vi "V1_moveby_commands_all.vi"(8 "error in (no error)":errorcluster, 9 "DAQ channel":tag, 10 "channel":i32(ring)=1 items=["Channel1"=1, "Channel2"=2, "Channel3"=3, "Channel4"=4], 11 ".NET Refnum in":refnum<k24>) -> (0 "error out":errorcluster, 3 ".NET Refnum out":refnum<k24>)   [LabVIEW 2020]
uses:
  C:/Users/359167/Documents/LabVIEW_ws/Thorlabs.MotionControl.KCube.InertialMotorCLI.dll
  Thorlabs.MotionControl.KCube.InertialMotorCLI.dll
  <vilib>/DAQmx/read.llb/DAQmx Read (Analog 1D Wfm NChan NSamp).vi
  <vilib>/Analysis/baseanly.llb/Mean (DBL).vi
  <vilib>/DAQmx/create/channels.llb/DAQmx Create Channel (AI-Voltage-Basic).vi
  <vilib>/DAQmx/configure/timing.llb/DAQmx Timing (Sample Clock).vi
  <vilib>/DAQmx/miscellaneous.llb/DAQmx Fill In Error Info.vi
  <vilib>/Analysis/NI_AALBase.lvlib
panel:
  out "x*y":dbl
  out "Sensor Sampling":waveform(dbl)[](graph)
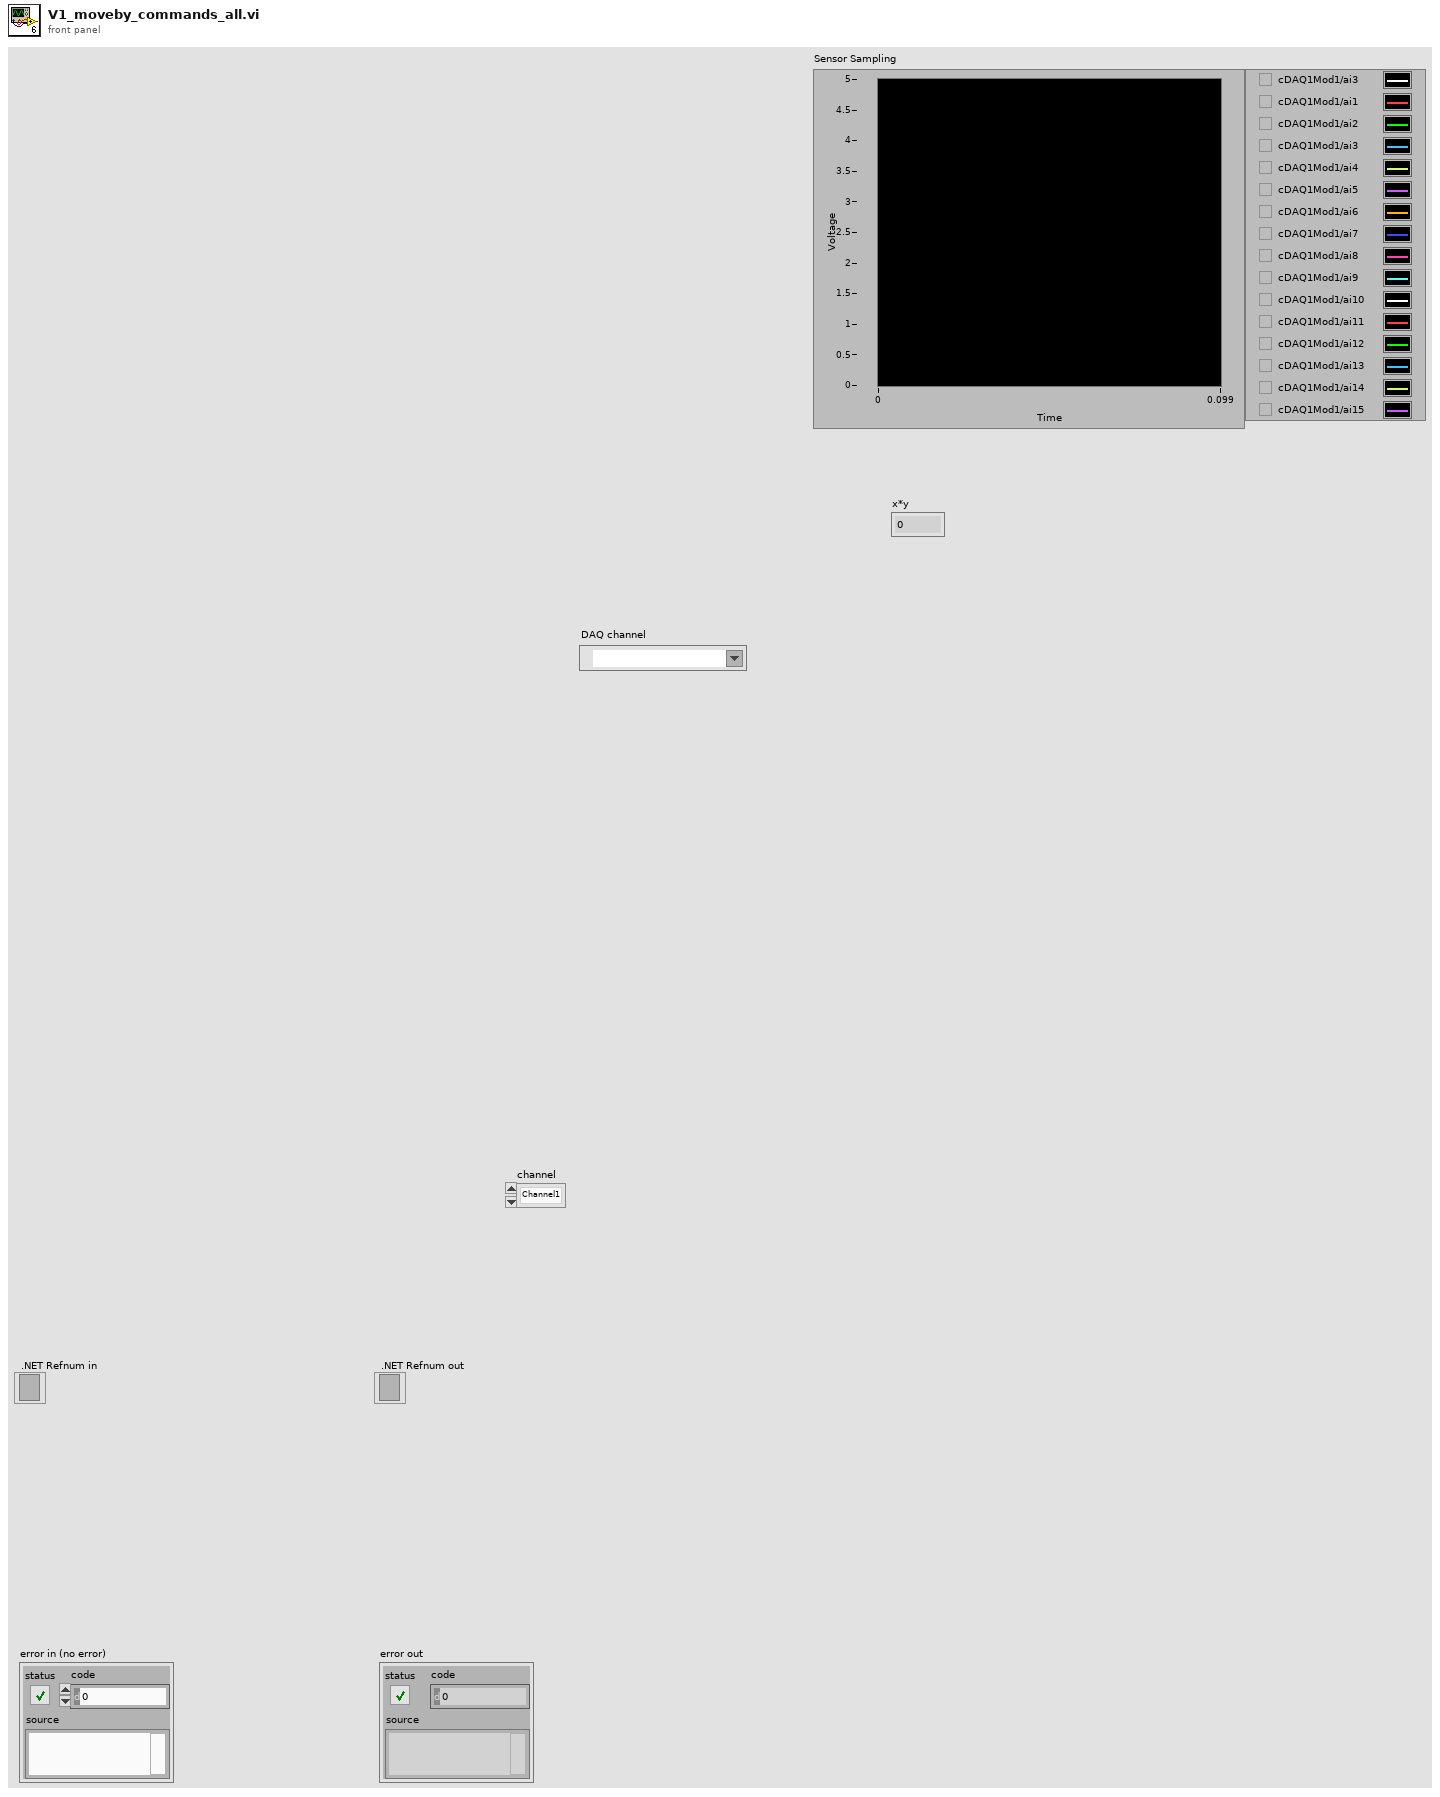
[diagram p1: front panel]
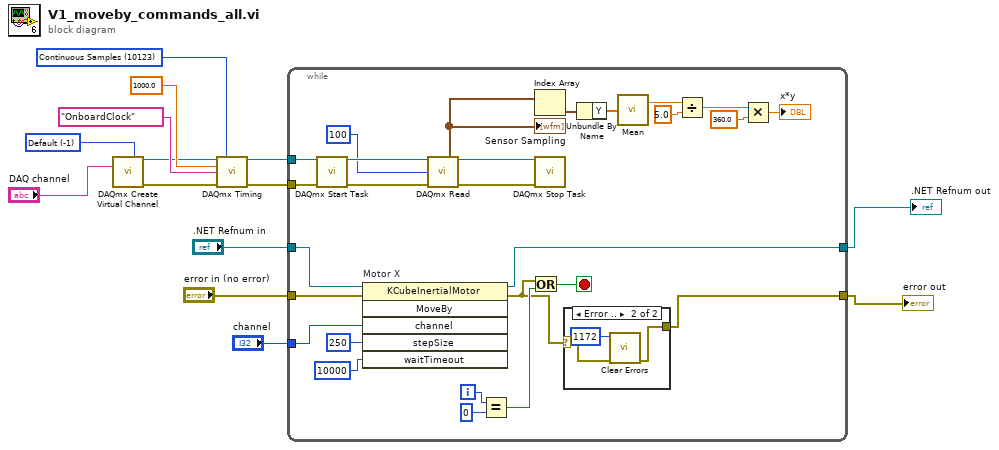
[diagram p0: block diagram]
diagram:
  w10 = -1 items=["Default"=-1, "RSE"=10083, "NRSE"=10078, "Differential"=10106, "Pseudodifferential"=12529] ("input terminal configuration")
  w11 = 10123 items=["Finite Samples"=10178, "Continuous Samples"=10123, "Hardware Timed Single Point"=12522] ("sample mode")
  n1 = call-poly <vilib>:"DAQmx Create Virtual Channel.vi"("input terminal configuration"=w10, "physical channels"="DAQ channel") -> ("task out"=w6:refnum<k21>, "error out"=w7:errorcluster)  [unwired: 12 in]
  n2 = call-poly <vilib>:"DAQmx Timing.vi"("task/channels in"=w6, "sample mode"=w11, "rate"=1000.0 ("sample rate"), "source"=tag "OnboardClock", "error in"=w7) -> ("task out"=w4:refnum<k21>, "error out"=w3:errorcluster)  [unwired: 9 in]
  n3 = while {
    tunnel: "channel" -> [w39]
    tunnel: w4 -> [w19]
    tunnel: w3 -> [w18]
    tunnel: ".NET Refnum in" -> [w33]
    tunnel: [w17] -> w1
    tunnel: "error in (no error)" -> [w37]
    tunnel: [w15] -> w2
    i -> [w34]
    stop <- w35 stop-if-true
    n4 = call <vilib>:"DAQmx Start Task.vi"("task/channels in"=w19, "error in"=w18) -> ("task out"=w29:refnum<k21>, "error out"=w30:errorcluster)  [unwired: 12 in]
    n5 = invoke on="Motor X" class="KCubeInertialMotor" method="MoveBy"(reference=w33, error in=w37, "channel"=w39, "stepSize"=250, "waitTimeout"=10000) -> (reference out=w17:refnum<k24>, error out=w16:errorcluster)  [unwired: 1 in, 4 out]
    n6 = call-poly <vilib>:"DAQmx Read.vi"("task/channels in"=w29, "number of samples per channel"=100 ("n samples/channel"), "error in"=w30) -> ("data"=w21:waveform(dbl)[], "task out"=w31:refnum<k21>, "error out"=w32:errorcluster)  [unwired: 10 in]
    "Sensor Sampling" <- w21
    n7 = Equal?(x=w34, y=0) -> (x = y?=w36:bool)
    n8 = Or(x=w16, y=w36) -> (x .or. y?=w35:bool)
    n9 = Index Array(array=w21) -> (element=w27:waveform(dbl))  [unwired: 1 in]
    n10 = call <vilib>:"DAQmx Stop Task.vi"("task/channels in"=w31, "error in"=w32) -> ()  [unwired: 12 in, 2 out]
    n11 = case shown="Error .." w16 {
      selector: w16 -> [w42 w44]
      tunnel: [w42 w43] -> w15
      frame No Error {
      }
      frame Error {
        n12 = call <vilib>:"Clear Errors.vi"("error in (no error)"=w44, "specific error code to clear (0: all)"=1172) -> ("error out"=w43:errorcluster)  [unwired: 4 in, 1 out]
      }
    }
    n13 = Unbundle By Name(w27) -> ("Y"=w26:dbl[])
    n14 = call-poly <vilib>:"Mean.vi"("X"=w26) -> ("mean"=w25:dbl)  [unwired: 1 out]
    n15 = Divide(x=w25, y=5.0) -> (x/y=w24:dbl)
    n16 = Multiply(x=w24, y=360.0) -> (x*y=→"x*y":dbl)
  }
  "error out" <- w2
  ".NET Refnum out" <- w1
